vi "Manage_Monitor.vi"   [LabVIEW 2016]
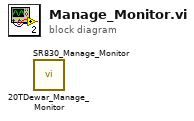
[diagram p0: block diagram]
diagram:
  n1 = call "20TDewar_Manage_Monitor.vi"() -> ()  [unwired: 6 in, 2 out]
  n2 = call "SR830_Manage_Monitor.vi"() -> ()  [unwired: 6 in, 2 out]
